vi "CC FITS Write Obs Data in FITS Header.vi"(8 "error in (no error)":errorcluster, 11 "gfits refnum":T1) -> (0 "error out":errorcluster, 3 "dup gfits refnum":T1)   [LabVIEW 2024]
uses:
  gfitsio/gfitsio-refnum.ctl
  gfitsio/gfitsio-write-key-string.vi
  gfitsio/gfitsio.lvlib
  Telescope/LDT Telescope/LDT Telescope.lvclass
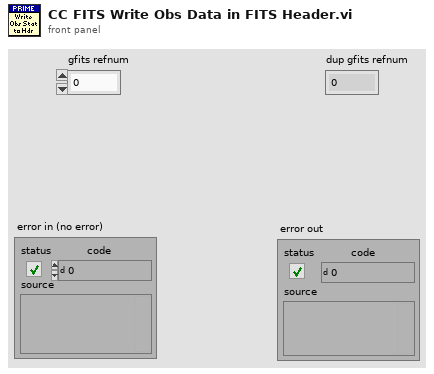
[diagram p1: front panel]
types:
  T1 = typedef "gfitsio.lvlib/gfitsio-refnum.ctl" = u64
  T2 = typedef "LDT Telescope.lvclass/LDT FITS Keyword cluster.ctl" = cluster{"Keyword":string, "Value":string, "Comment":string, "Valid":bool}
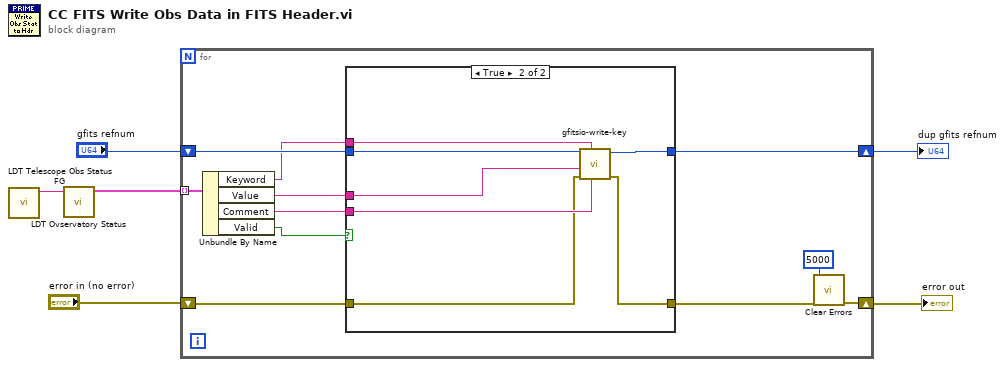
[diagram p0: block diagram]
diagram:
  n1 = call "LDT Telescope Obs Status FG.vi"() -> ("status string out"=w3:string)  [unwired: 10 in, 1 out]
  n2 = call "LDT Ovservatory Status.vi"("XML Locutus Obs Status String"=w3) -> ("keywords"=w2:T2[])  [unwired: 10 in]
  n3 = for {
    shift-right: [w16] -> w5
    shift-left: "gfits refnum" -> [w17]
    shift-right: [w15] -> w4
    shift-left: "error in (no error)" -> [w8]
    tunnel: w2 -> [w13] mode=indexing
    n4 = Unbundle By Name(w13) -> ("Keyword"=w11:string, "Value"=w10:string, "Comment"=w9:string, "Valid"=w12:bool)
    n5 = case shown="True" w12 {
      tunnel: w17 -> [w18 w26]
      tunnel: [w18 w25] -> w16
      tunnel: w11 -> [_ w24]
      tunnel: w10 -> [_ w23]
      tunnel: w9 -> [_ w22]
      tunnel: w8 -> [w19 w21]
      tunnel: [w19 w20] -> w7
      frame False {
      }
      frame True {
        n6 = call-poly "gfitsio-write-key.vi"("comment"=w22, "keyname"=w24, "error in (no error)"=w21, "value"=w23, "gfits refnum"=w26) -> ("error out"=w20:errorcluster, "dup gfits refnum"=w25:T1)  [unwired: 5 in]
      }
    }
    n7 = call <vilib>:"Clear Errors.vi"("error in (no error)"=w7, "specific error code to clear (0: all)"=5000) -> ("error out"=w15:errorcluster)  [unwired: 4 in, 1 out]
  }
  "error out" <- w4
  "dup gfits refnum" <- w5
